vi "servo and IR.vi"() -> ()   [LabVIEW 2016]
uses:
  <vilib>/imath/engines/lvmath/Plug In/_Char/NIMS_CH_character datatype.ctl
  <vilib>/myRIO/Common/Instrument Driver Framework/myRIO v1.0/UART/vis/myRIO v1.0 Close UART.vi
  <vilib>/imath/engines/lvmath/Plug In/_Char/NIMS_CH_Character 1D to U8 1D.vi
  <vilib>/imath/engines/lvmath2/RunTimeEngine/BuiltInFunctions/var/NIMS_var(GV,RV).vi
  <instcachedir>/0/NIMS_var(GV,RV)_4069E0180F614BA3BA7EF465AF0C1F39.lvgen/NIMS_var(GV,RV)_4069E0180F614BA3BA7EF465AF0C1F39_001.vi
  <vilib>/imath/engines/lvmath2/RunTimeEngine/ErrorHandling/NIMS_Error From Error Code.vi
  <vilib>/imath/engines/lvmath2/RunTimeEngine/VariableToken/NIMS_VariableToken_CondDefined.vi
  <instcachedir>/0/NIMS_VariableToken_CondDefined_06E9DA95BD4D46A6BA55EC651A891960.lvgen/NIMS_VariableToken_CondDefined_06E9DA95BD4D46A6BA55EC651A891960_004.vi
  <vilib>/imathl/engines/lvmath/Functions/Error Handling/Create Error.vi
  <vilib>/imath/engines/lvmath2/RunTimeEngine/NodeEndStatement/NIMS_NodeEndStatement_Output.vi
  <instcachedir>/0/NIMS_NodeEndStatement_Output_53EC0D466D134D7ABD903AC30B43404B.lvgen/NIMS_NodeEndStatement_Output_53EC0D466D134D7ABD903AC30B43404B_001.vi
  <vilib>/imath/engines/lvmath2/RunTimeEngine/ErrorHandling/NIMS_Finalize Error.vi
  <vilib>/myRIO/Common/Instrument Driver Framework/Utilities/vis/FPGA Ref Manager.vi
  <vilib>/myRIO/Common/Instrument Driver Framework/myRIO v1.0/myRIO v1.0 Reset FPGA.vi
  <vilib>/myRIO/Common/Instrument Driver Framework/myRIO v1.0/IRQ/vis/myRIO v1.0 IRQ Info FGV.vi
  <vilib>/myRIO/Common/Instrument Driver Framework/myRIO v1.0/IRQ/vis/myRIO v1.0 Timer IRQ Info FGV.vi
  <vilib>/myRIO/Common/Instrument Driver Framework/myRIO v1.0/IRQ/vis/myRIO v1.0 ISR Agent.vi
  <vilib>/myRIO/Instrument Drivers/Utilities/Utilities.lvlib
panel:
  in  "A/DIO":bool
  in  "B/DIO":bool
  out "PWM 2":dbl=0.5
  in  "stop":bool
  in  "Numeric Control":u32
  out "angle(offset)":dbl
  out "Range [cm]":dbl(knob) scale=0.0..170.0
  # "IR"
  # "SERVO CONTROL"
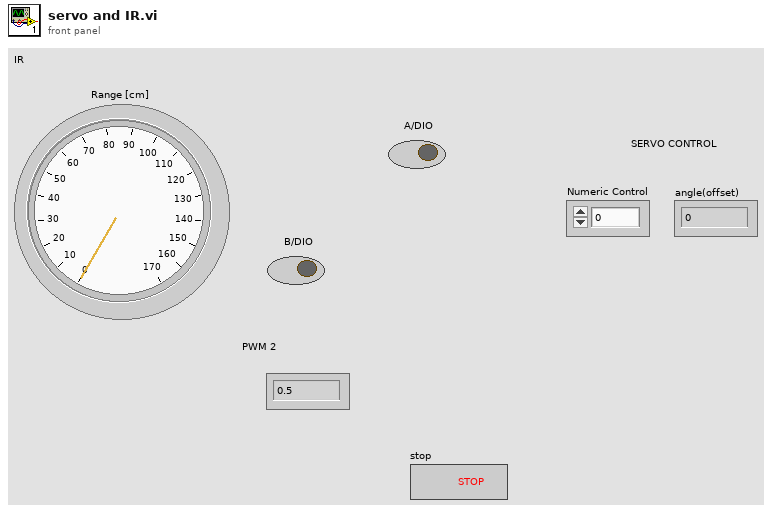
[diagram p1: front panel]
types:
  T1 = typedef "NIMS_CH_character datatype.ctl" = cluster{"Numeric":u8}
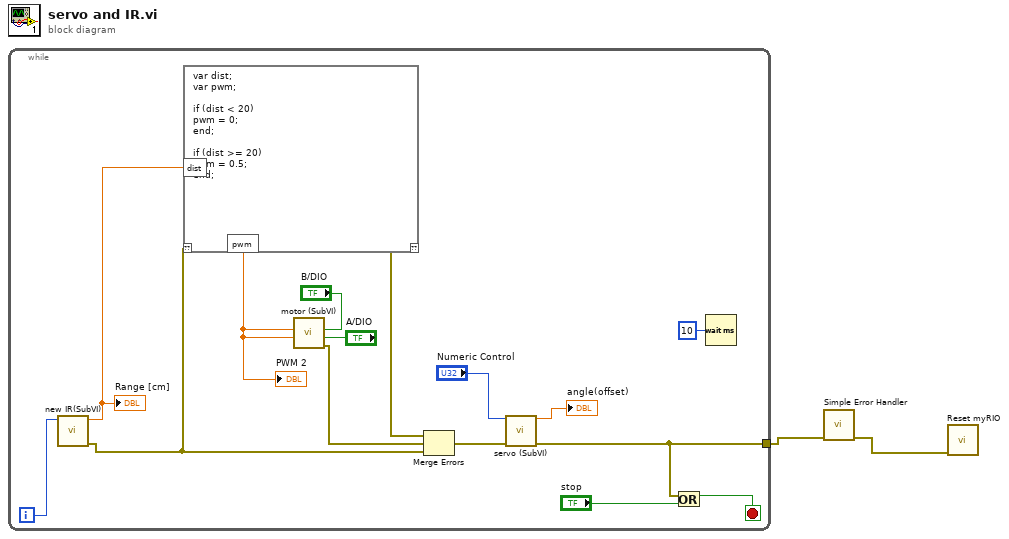
[diagram p0: block diagram]
diagram:
  n1 = while {
    tunnel: [w11] -> w1
    i -> [w13]
    stop <- w16 stop-if-true
    n2 = call "new IR(SubVI).vi"("Current"=w13) -> ("Range [cm] 2"=w5:dbl, "error out"=w3:errorcluster)  [unwired: 8 in]
    "Range [cm]" <- w5
    n3 = mathscript code="var dist;\nvar pwm;\n\nif (dist < 20)\npwm = 0;\nend;\n\nif (dist >= 20)\npwm = 0.5;\nend;"("??"=w3, "dist"=w5) -> ("??"=w6:errorcluster, "pwm"=w4:dbl)
    "PWM 2" <- w4
    n4 = call "motor (SubVI).vi"("PWM 2"=w4, "PWM 1"=w4, "B/DIO"="B/DIO", "A/DIO"="A/DIO") -> ("error out"=w7:errorcluster)  [unwired: 5 in]
    n5 = Merge Errors(w6, w7, w3) -> (w8:errorcluster)
    n6 = call "servo (SubVI).vi"("Numeric Control"="Numeric Control", "error in (no error)"=w8) -> ("angle(offset)"=→"angle(offset)":dbl, "error out"=w11:errorcluster)  [unwired: 12 in]
    n7 = Or(x=w11, y="stop") -> (x .or. y?=w16:bool)
    n8 = Wait (ms)(milliseconds to wait=u32 10) -> ()  [unwired: 1 out]
  }
  n9 = call <vilib>:"Simple Error Handler.vi"("error in (no error)"=w1) -> ("error out"=w2:errorcluster)  [unwired: 4 in, 4 out]
  n10 = call <vilib>:"Reset myRIO.vi"("error in (no error)"=w2) -> ()  [unwired: 10 in, 1 out]
